vi "QueryServer_GetRequest_AnalogInput.vi"(6 "error in (no error)":errorcluster, 9 "gRPCid":T3) -> (0 "error out":errorcluster, 3 "gRPCid out":T3)   [LabVIEW 2019, in "labview-grpc-query-server.lvlib"]
uses:
  labview-grpc-query-server.lvlib
  ea7aee44-32c1-4253-ac5d-59c6ef46377d.vi
  QueryServer_AnalogInputRequest.ctl
  VIs/grpcId.ctl
  VIs/gprc-support.lvlib
  QueryServer_DataTypeTest.ctl
  QueryServer_TestDataTypesParameters.ctl
panel:
  out "Request Data":T1
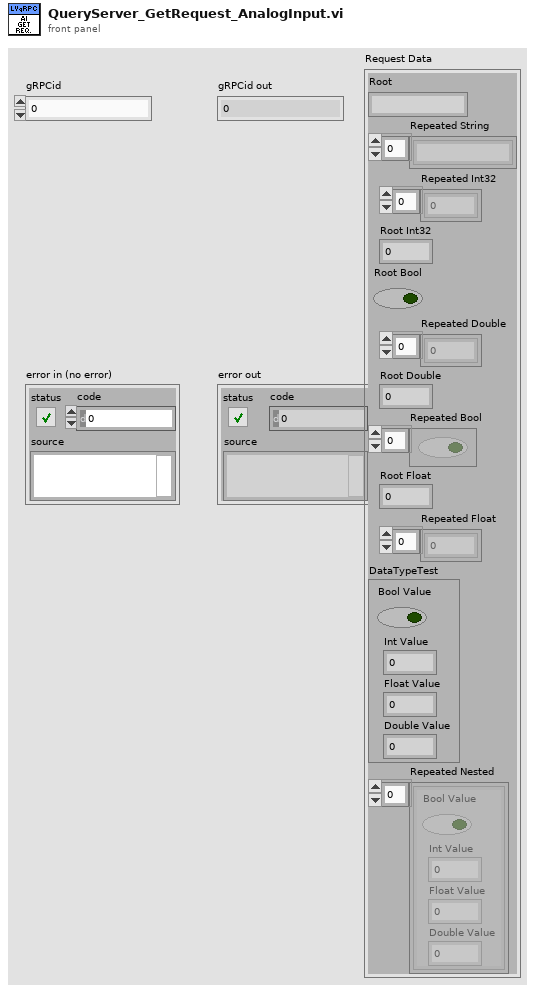
[diagram p1: front panel]
types:
  T1 = typedef "labview-grpc-query-server.lvlib/QueryServer_TestDataTypesParameters.ctl" = cluster{"Root":string, "Repeated String":string[], "Repeated Int32":i32[], "Root Int32":i32, "Root Bool":bool, "Repeated Double":dbl[], "Root Double":dbl, "Repeated Bool":bool[], "Root Float":sgl, "Repeated Float":sgl[], "DataTypeTest":T2, "Repeated Nested":T2[]}
  T2 = typedef "labview-grpc-query-server.lvlib/QueryServer_DataTypeTest.ctl" = cluster{"Bool Value":bool, "Int Value":i32, "Float Value":sgl, "Double Value":dbl}
  T3 = typedef "gprc-support.lvlib/grpcId.ctl" = u64
  T4 = typedef "QueryServer_AnalogInputRequest.ctl" = cluster{}
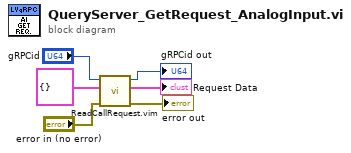
[diagram p0: block diagram]
diagram:
  n1 = call "ReadCallRequest.vim"("error in (no error)"="error in (no error)", "Data Type"=T4 {} ("AnalogInputRequest"), "gRPCid in"="gRPCid") -> ("error out"=→"error out":errorcluster, "Request Data"=→"Request Data":T1, "gRPCid out"=→"gRPCid out":T3)  [unwired: 6 in]
